vi "App_Queue Initialize.vi"(8 "error in":errorcluster) -> (0 "error out":errorcluster, 3 "Main Queue":T1)   [LabVIEW 2018, in "Application 1.lvlib"]
uses:
  Application 1.lvlib
  Data Def/App_Main Queue.ctl
  Data Def/App_Main Loop Queue Data.ctl
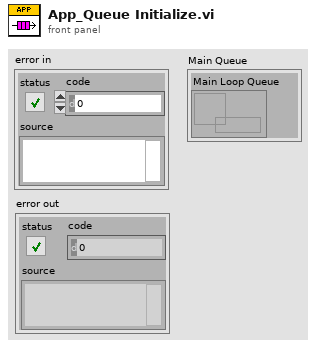
[diagram p1: front panel]
types:
  T1 = typedef "Application 1.lvlib/App_Main Queue.ctl" = cluster{"Main Loop Queue":refnum<queue>}
  T2 = typedef "Application 1.lvlib/App_Main Loop Queue Data.ctl" = cluster{"Command":string, "Data":variant}
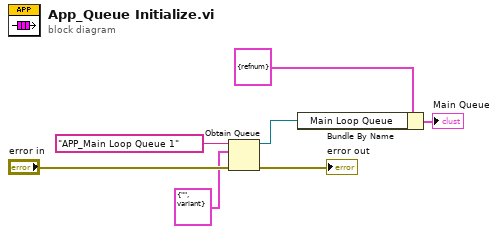
[diagram p0: block diagram]
diagram:
  n1 = Obtain Queue(name (unnamed)="APP_Main Loop Queue 1", element data type=T2 {"Command"="", "Data"=variant} ("Main Loop Queue Data"), error in (no error)="error in") -> (queue out=w3:refnum<queue>, error out=→"error out":errorcluster)  [unwired: 2 in, 1 out]
  n2 = Bundle By Name(cluster=T1 {"Main Loop Queue"=refnum} ("Main Queue"), "Main Loop Queue"=w3) -> (→"Main Queue":T1)
